vi "SN Gen.vi"(8 "error in (no error)":errorcluster, 9 "Date In":string, 10 "SN In":i32, 11 "PN In":string) -> (0 "error out":errorcluster, 1 "SN Out":string, 2 "Shift":string, 3 "Date":string)   [LabVIEW 2018]
panel:
  out "current time":timestamp
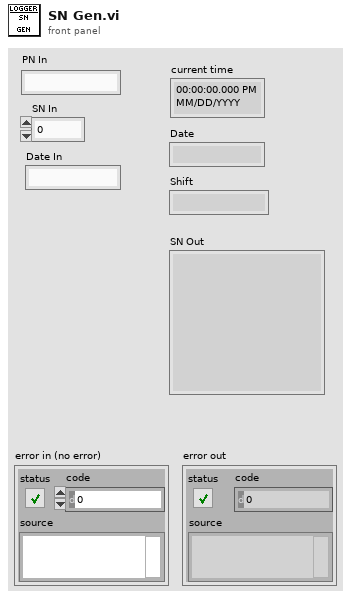
[diagram p1: front panel]
types:
  T1 = typedef "LVDateTimeRec.ctl" = cluster{"fractional second":dbl, "second":i32, "minute":i32, "hour":i32, "day of month":i32, "month":i32, "year":i32, "day of week":i32, "day of year":i32, "DST":i32}
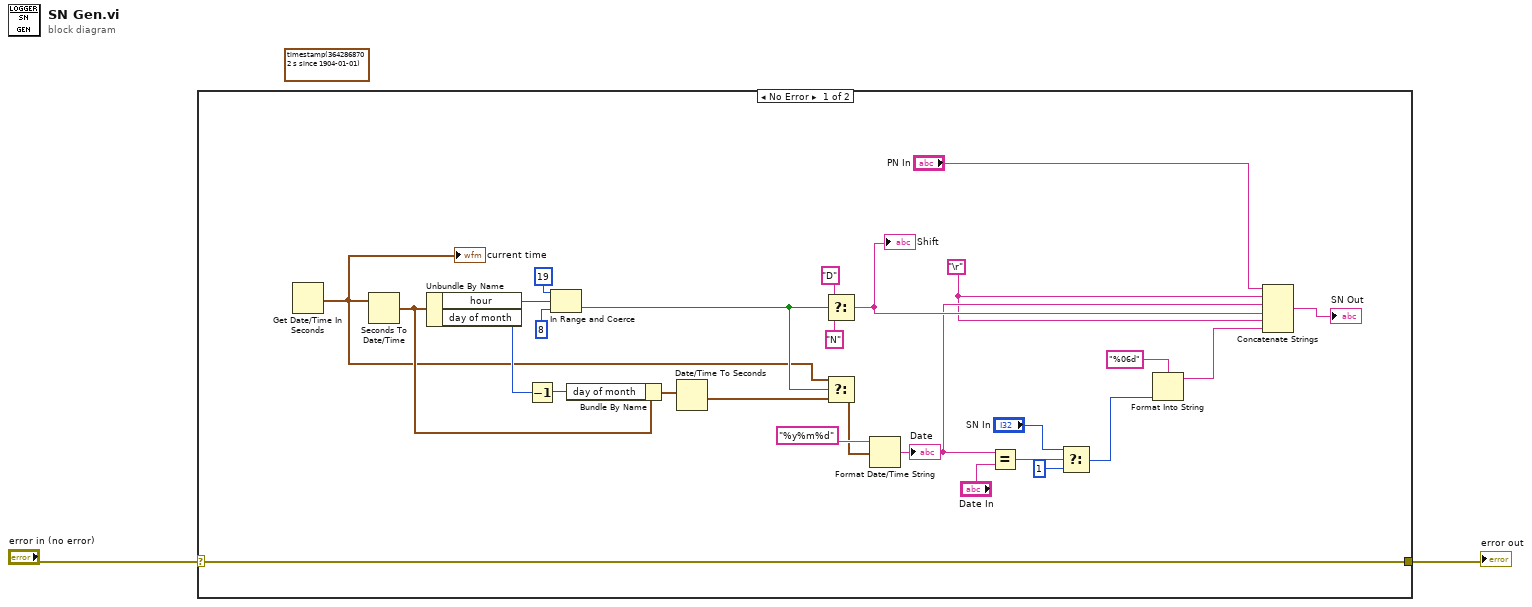
[diagram p0: block diagram]
diagram:
  (unwired) timestamp(3642868702.046 s since 1904-01-01) ("current time")
  n1 = case shown="No Error" "error in (no error)" {
    selector: "error in (no error)" -> [w11 w30]
    tunnel: [w11 w30] -> w1
    frame No Error {
      w3 = "\r"
      n2 = Get Date/Time In Seconds() -> (seconds since 1Jan1904=w13:timestamp)
      "current time" <- w13
      n3 = Seconds To Date/Time(time stamp (now)=w13) -> (date time rec=w17:T1)  [unwired: 1 in]
      n4 = Unbundle By Name(w17) -> ("hour"=w23:i32, "day of month"=w21:i32)
      n5 = Decrement(x=w21) -> (x-1=w24:i32)
      n6 = In Range and Coerce(upper limit=i16 19, x=w23, lower limit=i16 8 ("upper limit")) -> (In Range?=w20:bool)  [unwired: 1 out]
      n7 = Bundle By Name(cluster=w17, "day of month"=w24) -> (w22:T1)
      n8 = Date/Time To Seconds(2:w22) -> (0:w19:timestamp)  [unwired: 1 in]
      n9 = Select(t="D", s=w20, f="N") -> (s? t:f=w14:string)
      "Shift" <- w14
      n10 = Select(t=w13, s=w20, f=w19) -> (s? t:f=w18:timestamp)
      n11 = Format Date/Time String(time format string (%c)="%y%m%d", seconds (now)=w18) -> (date/time string=w10:string)  [unwired: 1 in]
      "Date" <- w10
      n12 = Equal?(x=w10, y="Date In") -> (x = y?=w8:bool)
      n13 = Select(t="SN In", s=w8, f=1) -> (s? t:f=w5:i32)
      n14 = Format Into String(format string="%06d", w5) -> (resulting string=w4:string)  [unwired: 2 in, 1 out]
      n15 = Concatenate Strings("PN In", w3, w10, w14, w3, w4) -> (→"SN Out":string)
    }
    frame Error {
    }
  }
  "error out" <- w1
